vi "FGV Actor Enqueuer.vi"(8 "Error In":errorcluster, 9 "Actor Enqueuer":refnum<class "Message Enqueuer.lvclass">, 10 "Actor Name":string, 11 "Action (read)":T1(ring)=enum."read") -> (0 "Error Out":errorcluster, 1 "Actor Enqueuer":refnum<class "Message Enqueuer.lvclass">, 2 "Success":bool, 4 "Actor Names":string[](array[string]), 6 "Actor Enqueuers":refnum<class "Message Enqueuer.lvclass">[](array[class]))   [LabVIEW 2012, in "CS++Base.lvlib"]
doc: "This is a FGV to be used to maintain a list of actor enqueuers."
uses:
  CS++Base.lvlib
  <vilib>/ActorFramework/Message Enqueuer/Message Enqueuer.lvclass
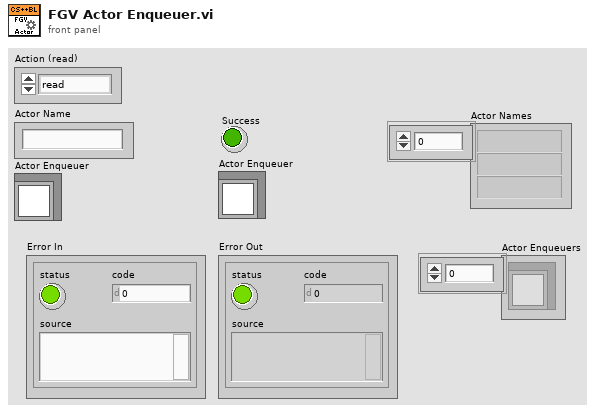
[diagram p1: front panel]
types:
  T1 = enum16{"add", "replace", "read", "remove", "reset", "get attibutes", ""}
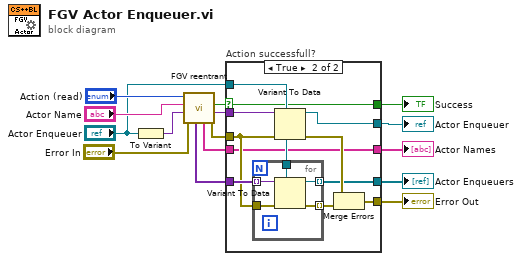
[diagram p0: block diagram]
diagram:
  n1 = To Variant(anything="Actor Enqueuer") -> (Variant=w12:variant)
  n2 = call "FGV reentrant.vi"("Error In"="Error In", "Data"=w12, "Attribute Name"="Actor Name", "Action (read)"="Action (read)") -> ("Error Out"=w8:errorcluster, "Data"=w11:variant, "Success"=w3:bool, "Attributes"=w4:string[], "values"=w9:variant[])  [unwired: 3 in]
  n3 = case "Action successfull?" shown="True" w3 {
    selector: w3 -> [w17 w19]
    tunnel: w11 -> [_ w28]
    tunnel: "Actor Enqueuer" -> [_ w27]
    tunnel: w9 -> [_ w26]
    tunnel: w8 -> [w16 w25]
    tunnel: [w16 w22] -> w7
    tunnel: [_ w21] -> w6
    tunnel: [_ w20] -> w5
    tunnel: w4 -> [_ w20]
    tunnel: [w17 w19] -> w2
    tunnel: [_ w18] -> w1
    frame False {
    }
    frame True {
      n4 = for {
        tunnel: w27 -> [w33]
        tunnel: w26 -> [w32] mode=indexing
        tunnel: w25 -> [w31]
        tunnel: [w30] -> w24 mode=indexing
        tunnel: [w29] -> w21 mode=indexing
        n5 = Variant To Data(error in=w31, type=w33, Variant=w32) -> (data=w29:refnum<class "Message Enqueuer.lvclass">, error out=w30:errorcluster)
      }
      n6 = Variant To Data(error in=w25, type=w27, Variant=w28) -> (data=w18:refnum<class "Message Enqueuer.lvclass">, error out=w23:errorcluster)
      n7 = Merge Errors(w23, w24) -> (w22:errorcluster)
    }
  }
  "Error Out" <- w7
  "Actor Names" <- w5
  "Actor Enqueuers" <- w6
  "Success" <- w2
  "Actor Enqueuer" <- w1
